vi "TEST Get Wind Speeds - Solution.vi"() -> ()   [LabVIEW 2009]
doc: "Two VI solution that allows the user to test the Wind Turbine class. Speed is set in one VI and read in another.\n\nAAL 9/09"
uses:
  SEQ - Solution.lvlib
panel:
  in  "Exit":bool
  out "Turbines":dbl[](array[numeric])
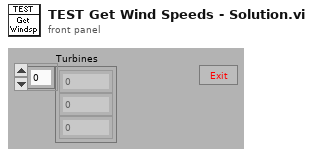
[diagram p1: front panel]
types:
  T1 = typedef "SEQ - Solution.lvlib/Wind Turbine DataRef.ctl" = refnum<queue>
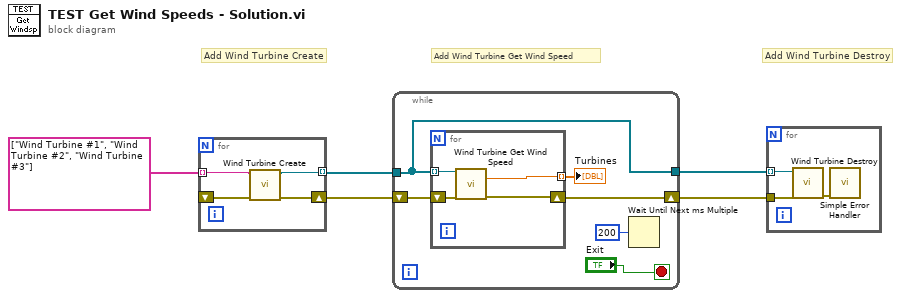
[diagram p0: block diagram]
diagram:
  # "Add Wind Turbine Destroy"
  # "Add Wind Turbine Get Wind Speed"
  # "Add Wind Turbine Create"
  n1 = for {
    tunnel: string[] ["Wind Turbine #1", "Wind Turbine #2", "Wind Turbine #3"] -> [w9] mode=indexing
    tunnel: [w8] -> w4 mode=indexing
    shift-right: [w6] -> w2
    shift-left: _ -> [w7]
    n2 = call "Wind Turbine Create.vi"("error in (no error)"=w7, "SEQ Name"=w9) -> ("error out"=w6:errorcluster, "Data Refnum out"=w8:T1)  [unwired: 8 in]
  }
  n3 = while {
    tunnel: w4 -> [w14]
    tunnel: [w14] -> w3
    shift-right: [w10] -> w1
    shift-left: w2 -> [w11]
    stop <- "Exit" stop-if-true
    n4 = for {
      tunnel: w14 -> [w19] mode=indexing
      tunnel: [w17] -> w15 mode=indexing
      shift-right: [w16] -> w10
      shift-left: w11 -> [w18]
      n5 = call "Wind Turbine Get Wind Speed.vi"("Data Refnum"=w19, "error in (no error)"=w18) -> ("Wind Speed (M/s)"=w17:dbl, "error out"=w16:errorcluster)  [unwired: 11 in, 1 out]
    }
    "Turbines" <- w15
    n6 = Wait Until Next ms Multiple(millisecond multiple=u32 200) -> ()  [unwired: 1 out]
  }
  n7 = for {
    tunnel: w3 -> [w22] mode=indexing
    tunnel: w1 -> [w21]
    n8 = call "Wind Turbine Destroy.vi"("error in (no error)"=w21, "Data Refnum"=w22) -> ("error out"=w20:errorcluster)  [unwired: 8 in, 1 out]
    n9 = call <vilib>:"Simple Error Handler.vi"("error in (no error)"=w20) -> ()  [unwired: 1 in, 8 out]
  }
